vi "Save McP ScanArray.dat V1.00.vi"(2 "McP ScanArray.dat Path":path, 3 "ScanPattern?":bool, 4 "ScanPattern":string="300.123\r400.123\r500.123\r600.123\r300.123\r400.123\r500.123\r600.123\r300.123\r400.123\r500.123\r600.123\r", 5 "format (%.3f)":string="%.3f", 6 "1D data":sgl[](array[numeric])=[700.1234, 800.1234, 900.1234, 1000.1235] format="%.5f") -> ()   [LabVIEW 2019]
uses:
  <vilib>/Utility/file.llb/Write To Spreadsheet File (DBL).vi
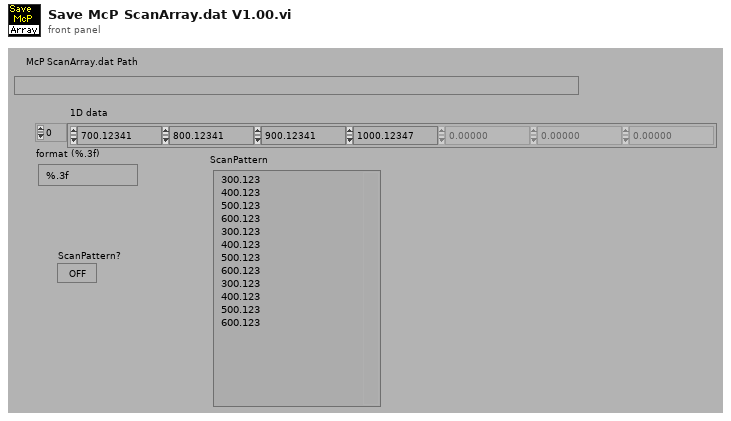
[diagram p1: front panel]
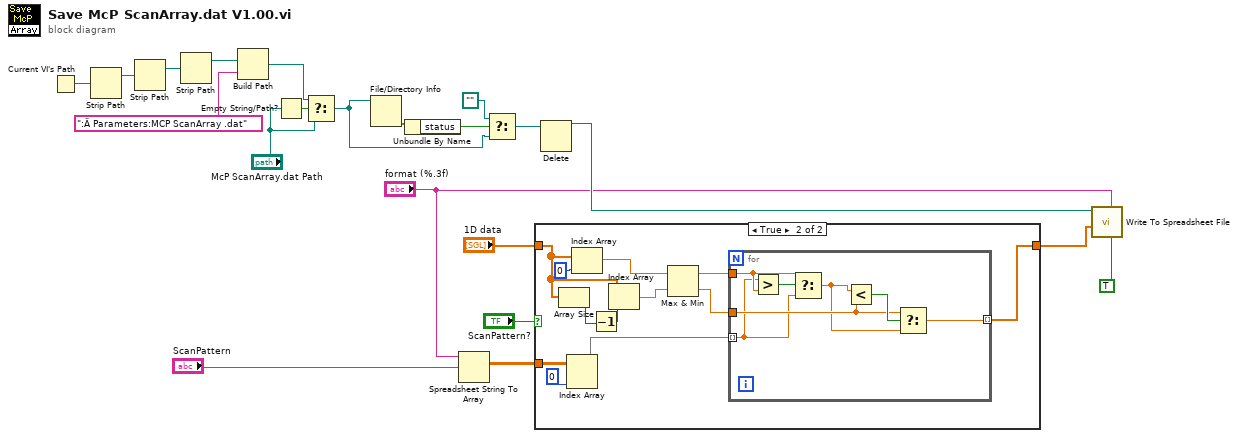
[diagram p0: block diagram]
diagram:
  n1 = Current VI's Path() -> (path=w13:path)
  n2 = Strip Path(path=w13) -> (stripped path=w17:path)  [unwired: 1 out]
  n3 = Strip Path(path=w17) -> (stripped path=w16:path)  [unwired: 1 out]
  n4 = Strip Path(path=w16) -> (stripped path=w14:path)  [unwired: 1 out]
  n5 = Build Path(base path=w14, name or relative path=":Ä Parameters:MCP ScanArray .dat") -> (appended path=w12:path)
  n6 = Empty String/Path?(string/path="McP ScanArray.dat Path") -> (empty?=w18:bool)
  n7 = Select(t=w12, s=w18, f="McP ScanArray.dat Path") -> (s? t:f=w10:path)
  n8 = File/Directory Info(path=w10) -> (error out=w21:errorcluster)  [unwired: 1 in, 6 out]
  n9 = Unbundle By Name(w21) -> ("status"=w20:bool)
  n10 = Spreadsheet String To Array(format string="format (%.3f)", spreadsheet string="ScanPattern") -> (array=w1:dbl[][])  [unwired: 2 in]
  n11 = Select(t=path "", s=w20, f=w10) -> (s? t:f=w8:path)
  n12 = case shown="True" "ScanPattern?" {
    tunnel: [w22 w23] -> w2
    tunnel: "1D data" -> [w22 w32]
    tunnel: w1 -> [_ w34]
    frame False {
    }
    frame True {
      n13 = Array Size(array=w32) -> (size(s)=w30:i32)
      n14 = Index Array(array=w34, index (col)=0 ("Index")) -> (element=w24:dbl[])  [unwired: 1 in]
      n15 = Index Array(array=w32, index=0 ("Index")) -> (element=w28:sgl)
      n16 = Decrement(x=w30) -> (x-1=w29:i32)
      n17 = Index Array(array=w32, index=w29) -> (element=w27:sgl)
      n18 = Max & Min(x=w28, y=w27) -> (max(x,y)=w26:sgl, min(x,y)=w25:sgl)
      n19 = for {
        tunnel: w26 -> [w40]
        tunnel: w25 -> [w38]
        tunnel: w24 -> [w36] mode=indexing
        tunnel: [w37] -> w23 mode=indexing
        n20 = Greater?(x=w36, y=w40) -> (0:w41:bool)
        n21 = Select(t=w40, s=w41, f=w36) -> (s? t:f=w35:dbl)
        n22 = Less?(x=w35, y=w38) -> (x < y?=w39:bool)
        n23 = Select(t=w38, s=w39, f=w35) -> (s? t:f=w37:dbl)
      }
    }
  }
  n24 = Delete(path (use dialog)=w8) -> (deleted path=w7:path)  [unwired: 4 in, 2 out]
  n25 = call-poly <vilib>:"Write To Spreadsheet File.vi"("transpose? (no:F)"=TRUE, "format (%.3f)"="format (%.3f)", "1D data"=w2, "file path (dialog if empty)"=w7) -> ()  [unwired: 4 in, 1 out]
